vi "Configure Mode.vi"(7 "Channel (1:Chan A)":i32(ring)=1 items=["System (To)", "Channel A", "Channel B", "Channel C", "Channel D", "Channel E", "Channel F", "Channel G", "Channel H"], 8 "error in (no error)":errorcluster, 10 "Mode (0:Normal)":T1(ring), 11 "VISA resource name":refnum<visa-resource-name>) -> (0 "error out":errorcluster, 3 "VISA resource name out":refnum<visa-resource-name>)   [LabVIEW 2012, in "Berkeley Nucleonics 500 Series.lvlib"]
doc: "This VI is used to configure the operating mode of the selected channel or system (To) timer."
uses:
  Berkeley Nucleonics 500 Series.lvlib
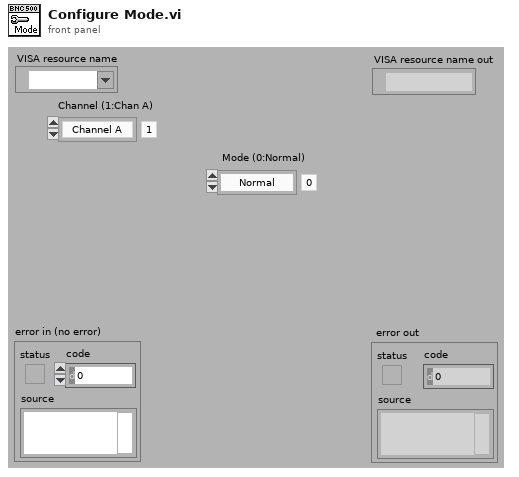
[diagram p1: front panel]
types:
  T1 = enum16{"Normal", "Single", "Burst", "Duty Cycle"}
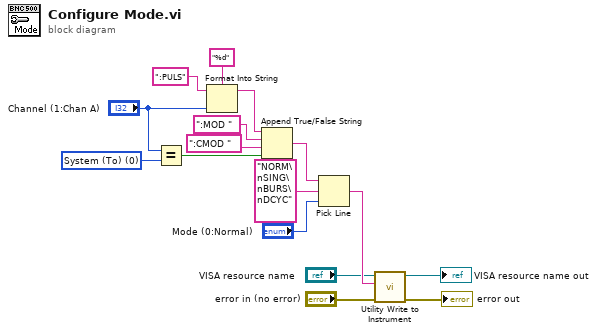
[diagram p0: block diagram]
diagram:
  w6 = 0 items=["System (To)", "Channel A", "Channel B", "Channel C", "Channel D", "Channel E", "Channel F", "Channel G", "Channel H"] ("Channel (1:Chan A)")
  n1 = Equal?(x="Channel (1:Chan A)", y=w6) -> (x = y?=w5:bool)
  n2 = Format Into String(format string="%d", initial string=":PULS", "Channel (1:Chan A)") -> (resulting string=w2:string)  [unwired: 1 in, 1 out]
  n3 = Append True/False String(1:w5, 2:":CMOD ", 3:":MOD ", 4:w2) -> (0:w1:string)
  n4 = Pick Line(string ("")=w1, multi-line string="NORM\nSING\nBURS\nDCYC", line index="Mode (0:Normal)") -> (output string=w16:string)
  n5 = call "Utility Write to Instrument.vi"("error in (no error)"="error in (no error)", "Write Buffer"=w16, "VISA resource name"="VISA resource name") -> ("error out"=→"error out":errorcluster, "VISA resource name out"=→"VISA resource name out":refnum<visa-resource-name>)  [unwired: 7 out]
